vi "VIPM Install VI Packages By Name.vi"   [LabVIEW 2016, in "Script.lvlib"]
uses:
  Script.lvlib
  <vilib>/Wiresmith Technology/G CLI/Argument Parser/Option Class/Option Configuration.ctl
  <vilib>/Wiresmith Technology/G CLI/Argument Parser/Option Class/Argument Type.ctl
  <vilib>/Wiresmith Technology/G CLI/CLI Class/CLI.lvclass
  <vilib>/Wiresmith Technology/G CLI/Argument Parser/Option Class/Option.lvclass
  <vilib>/Wiresmith Technology/G CLI/Argument Parser/Option Set Class/Option Set.lvclass
  <vilib>/JKI/VIPM API/VIPM API_vipm_api.lvlib
types:
  T1 = typedef "Option Parser.lvlib/Option.lvclass/Option Configuration.ctl" = cluster{"Option Type":T2, "Option Labels":string[], "Key":string, "Description":string, "Required":bool, "Default Value":string}
  T2 = typedef "Option Parser.lvlib/Option.lvclass/Argument Type.ctl" = enum16{"flag", "value"}
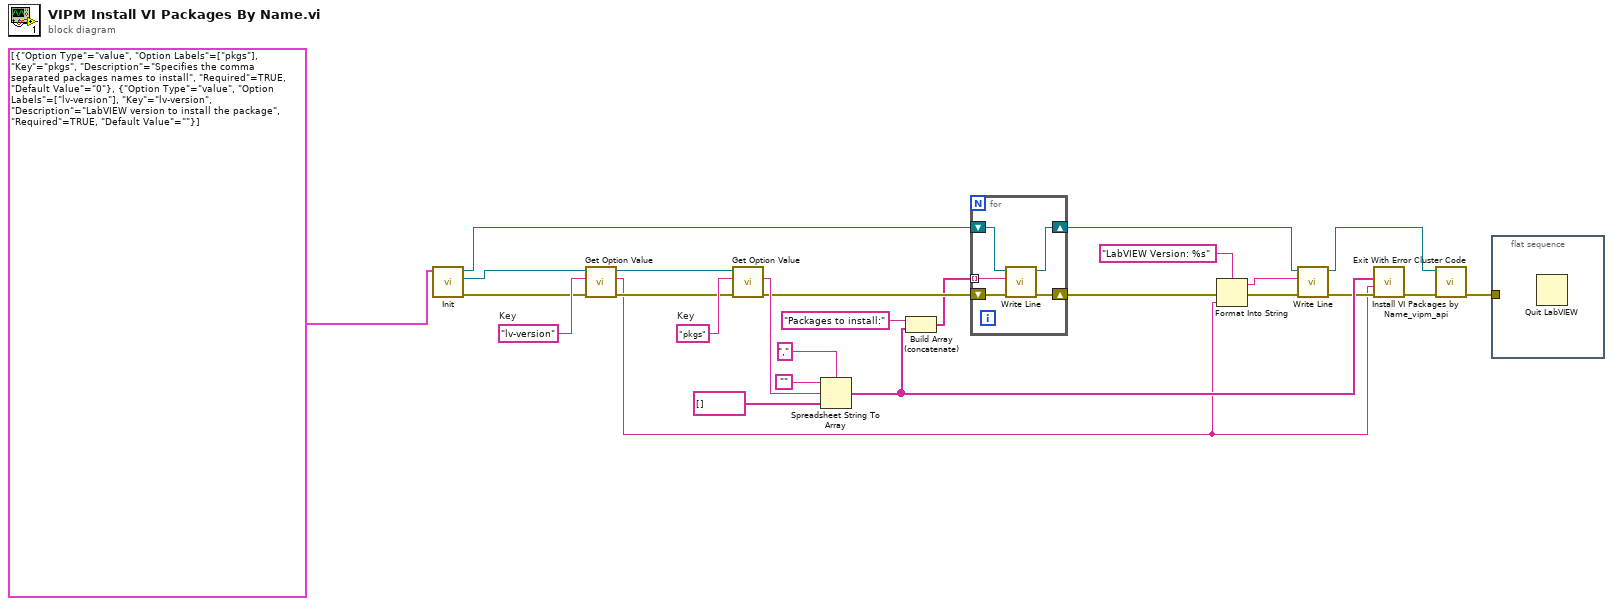
[diagram p0: block diagram]
diagram:
  w21 = "lv-version"  # Key
  w26 = "pkgs"  # Key
  n1 = call "Init.vi"("Options"=T1[] [{"Option Type"=enum."value", "Option Labels"=["pkgs"], "Key"="pkgs", "Description"="Specifies the comma separated packages names to install", "Required"=TRUE, "Default Value"="0"}, {"Option Type"=enum."value", "Option Labels"=["lv-version"], "Key"="lv-version", "Description"="LabVIEW version to install the package", "Required"=TRUE, "Default Value"=""}]) -> ("error out"=w4:errorcluster, "Option Set out"=w3:refnum<class "Option Set.lvclass">, "CLI out"=w2:refnum<class "CLI.lvclass">)  [unwired: 8 in]
  n2 = call <vilib>:"Get Option Value.vi"("error in (no error)"=w4, "Option Key"=w21, "Option Set in"=w3) -> ("error out"=w20:errorcluster, "Value"=w6:string, "Option Set out"=w19:refnum<class "Option Set.lvclass">)  [unwired: 5 in, 1 out]
  n3 = call <vilib>:"Get Option Value.vi"("error in (no error)"=w20, "Option Key"=w26, "Option Set in"=w19) -> ("error out"=w16:errorcluster, "Value"=w18:string)  [unwired: 5 in, 2 out]
  n4 = Spreadsheet String To Array(delimiter (Tab)=",", format string="", spreadsheet string=w18, array type (2D Dbl)=string[] [] ("Value")) -> (array=w14:string[])
  n5 = Build Array (concatenate)("Packages to install:" ("delimiter (Tab)"), w14) -> (w13:string[])
  n6 = for {
    shift-right: [w29] -> w11
    shift-left: w2 -> [w31]
    shift-right: [w30] -> w9
    shift-left: w16 -> [w28]
    tunnel: w13 -> [w27] mode=indexing
    n7 = call <vilib>:"Write Line.vi"("error in (no error)"=w28, "Text to Write"=w27, "CLI in"=w31) -> ("error out"=w30:errorcluster, "CLI out"=w29:refnum<class "CLI.lvclass">)  [unwired: 7 in]
  }
  n8 = Format Into String(format string="LabVIEW Version: %s" ("delimiter (Tab)"), error in=w9, w6) -> (resulting string=w5:string, error out=w8:errorcluster)  [unwired: 1 in]
  n9 = call <vilib>:"Write Line.vi"("error in (no error)"=w8, "Text to Write"=w5, "CLI in"=w11) -> ("error out"=w12:errorcluster, "CLI out"=w10:refnum<class "CLI.lvclass">)  [unwired: 7 in]
  n10 = call <vilib>:"Install VI Packages by Name_vipm_api.vi"("error in (no error)"=w12, "LabVIEW Version"=w6, "Package Names to Install []"=w14) -> ("error out"=w24:errorcluster)  [unwired: 8 in]
  n11 = call <vilib>:"Exit With Error Cluster Code.vi"("error in (no error)"=w24, "CLI in"=w10) -> ("error out"=w25:errorcluster)  [unwired: 9 in]
  n12 = flat-sequence {
    tunnel: w25 -> [_]
    frame #0 {
      n13 = Quit LabVIEW() -> ()  [unwired: 1 in]
    }
  }
